vi "Donut Plot Example.vi"() -> ()   [LabVIEW 2019]
uses:
  Python Visualizations Library/pieplot_labels.ctl
  Python Visualizations Library/Python Visualizations.lvlib
panel:
  in  "Donut Plot Title":string="My Donut Plot"
  in  "Dataset labels":string[](array[string])=["Pass", "Fail", "Error"]
  out "Donut Plot":picture
  in  "Plot Colors":u32[](array[colorbox])=[5898115, 16743234, 12698049]
  in  "Datasets":dbl[](array[numeric])=[50.0, 4.0, 2.0]
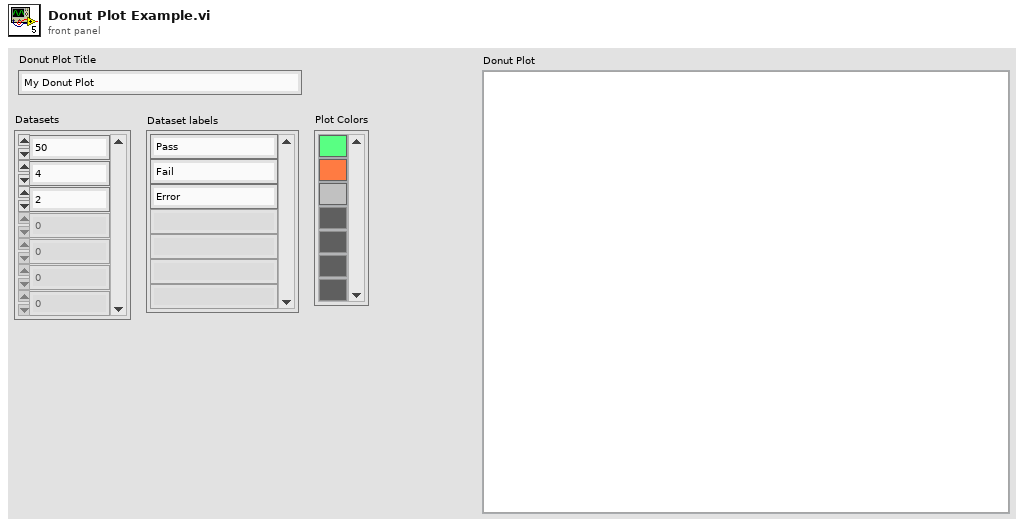
[diagram p1: front panel]
types:
  T1 = typedef "Python Visualizations.lvlib/pieplot_labels.ctl" = cluster{"dataset labels":string[], "title":string}
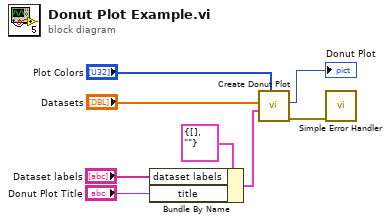
[diagram p0: block diagram]
diagram:
  n1 = Bundle By Name(cluster=T1 {"dataset labels"=[], "title"=""} ("labels"), "dataset labels"="Dataset labels", "title"="Donut Plot Title") -> (w1:T1)
  n2 = call "Create Donut Plot.vi"("plot colors"="Plot Colors", "labels"=w1, "datasets"="Datasets") -> ("error out"=w5:errorcluster, "donut plot"=→"Donut Plot":picture)  [unwired: 7 in]
  n3 = call <vilib>:"Simple Error Handler.vi"("error in (no error)"=w5) -> ()  [unwired: 4 in, 5 out]
